vi "Exponential Fit PtByPt.vi"(0 "y":dbl format="%0.2f", 1 "initialize":bool, 7 "x":dbl format="%0.2f", 11 "sample length":i32=100) -> (4 "Best Exponential Fit":dbl[](array[numeric]), 6 "amplitude":dbl format="%0.2f", 8 "damping":dbl format="%0.2f", 10 "mse":dbl format="%0.2f", 15 "error":i32)   [LabVIEW 2017, in "NI_PtbyPt.lvlib"]
doc: "Finds the exponential curve values and the exponential coefficients <B>amplitude</B> and <B>damping</B>, using the least-squares solution, which describe the exponential curve that best represents the input set of data points defined by <B>sample length</B>."
uses:
  <vilib>/ptbypt/NI_PtbyPt.lvlib
  <vilib>/Analysis/NI_AALPro.lvlib
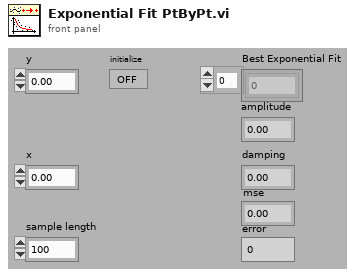
[diagram p1: front panel]
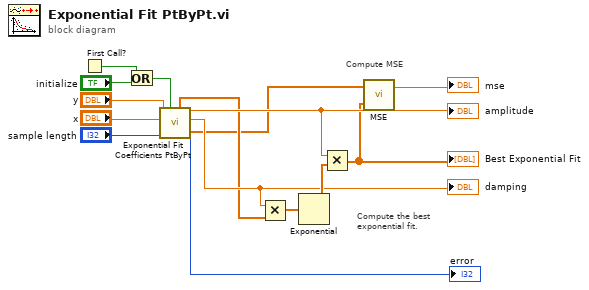
[diagram p0: block diagram]
diagram:
  # "Compute the best\nexponential fit."
  # "Compute MSE"
  n1 = First Call?() -> (First Call?: T/F=w1:bool)
  n2 = Or(x=w1, y="initialize") -> (x .or. y?=w3:bool)
  n3 = call <vilib>:"Exponential Fit Coefficients PtByPt.vi"("y"="y", "x"="x", "sample length"="sample length", "initialize"=w3) -> ("History of x"=w7:dbl[], "History of y"=w6:dbl[], "amplitude"=w11:dbl, "damping"=w12:dbl, "error"=→"error":i32)  [unwired: 2 in]
  "damping" <- w12
  "amplitude" <- w11
  n4 = Multiply(x=w12, y=w7) -> (x*y=w13:dbl[])
  n5 = Exponential(1:w13) -> (0:w14:dbl[])
  n6 = Multiply(x=w11, y=w14) -> (x*y=w9:dbl[])
  "Best Exponential Fit" <- w9
  n7 = call <vilib>:"MSE.vi"("X Values"=w9, "Y Values"=w6) -> ("mse"=→"mse":dbl)  [unwired: 1 out]
